vi "PrepareRollToPassRollerGoToTactic.vi"(7 "first call":bool, 8 "error in (no error)":errorcluster, 9 "Robot":refnum<class "Robot.lvclass">, 10 "Game in":refnum<class "Game.lvclass">, 11 "PrepareRollToPassRollerGoToTactic in":refnum<class "PrepareRollToPassRollerGoToTactic.lvclass">) -> (0 "error out":errorcluster, 2 "Robot out":refnum<class "Robot.lvclass">, 3 "PrepareRollToPassRollerGoToTactic out":refnum<class "PrepareRollToPassRollerGoToTactic.lvclass">)   [LabVIEW 2023, in "PrepareRollToPassRollerGoToTactic.lvclass"]
uses:
  PrepareRollToPassRollerGoToTactic.lvclass
  Robot_class/Robot.lvclass
  Game_class/Game.lvclass
  Robot_class/tactics.ctl
  Tactic_class/Tactic.lvclass/Tactic.ctl
  Skillbook_class/Skillbook.lvclass/Skillbook.ctl
  Robot_class/Robot.lvclass/Robot.ctl
  Object_class/Object.lvclass/Object.ctl
  Game_class/Game.lvclass/Game.ctl
  Parameters_class/Parameters.lvclass/Parameters.ctl
  Team_class/Team.lvclass/Team.ctl
  PrepareRollToPassRollerGoToTactic.lvclass/PrepareRollToPassRollerGoToTactic.ctl
  <vilib>/Analysis/_algsub.llb/Real Vector Norm.vi
  Game_class/Read Parameters.lvclass.vi
  Game_class/Read Utilities.lvclass.vi
  Game_class/Read OffensiveTeam.vi
  Team_class/Read RobotRef.vi
  Parameters_class/Read AttakingOurselves.vi
  Game_class/Read BallRef.vi
  Object_class/Read x.vi
  Object_class/Read y.vi
  Robot_class/Read id.vi
  Skillbook_class/Read GoToSkill.vi
  Tactic_class/Read Skillbook.vi
  Robot_class/Write tactic.vi
  Write States.vi
  Ball_class/Ball.lvclass
  Ally_class/Ally.lvclass
  Skillbook_class/Skillbook.lvclass
  Parameters_class/Parameters.lvclass
  Utilities_class/Utilities.lvclass
  GoToSkill_class/GoToSkill.lvclass
  <vilib>/Analysis/NI_AALPro.lvlib
panel:
  out "x .or. y?":bool
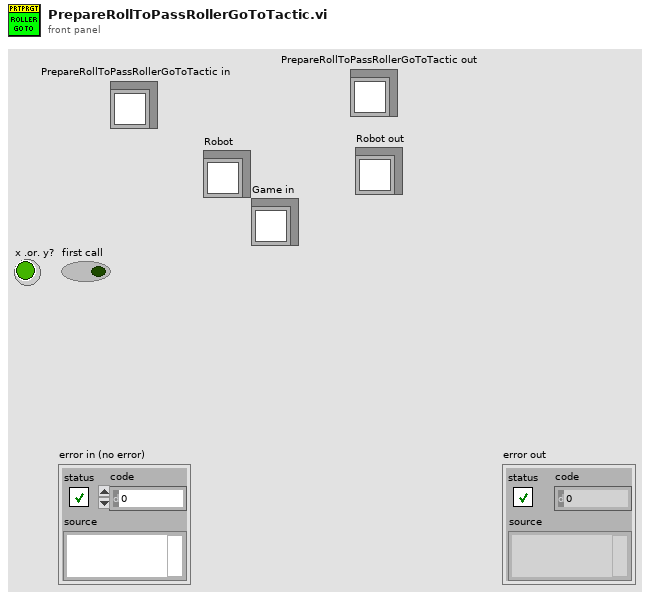
[diagram p1: front panel]
types:
  T1 = typedef "tactics.ctl" = enum16{"ReceivePassInFuturePoint", "Roller", "PrepareRollToPassRollerGoTo", "PrepareRollToPassReceiverGoTo", "WaitRoll", "PositionToRoll", "PenaltyAttacker", "PassObserver", "PenaltyDefense", "TableReceiverTactic", "Test", "DefendGoal", "Marker", "FollowAttacker", "DefendArea", "Shoot", "AttackerAimGoal", "AttackerBallOutOfField", "AttackerBlock", "AttackerStop", "Duelist", "Halt", "ZigZag", "GoTo", "Timeout", "KickToPassReceiver", "PositionToReceivePass", "DefendAreaVSS", "DefendGoalVSS", "KickVSS", "AttackVSS", "DispBallVSS", "PenaltyAttackVSS", "WaitPass"}
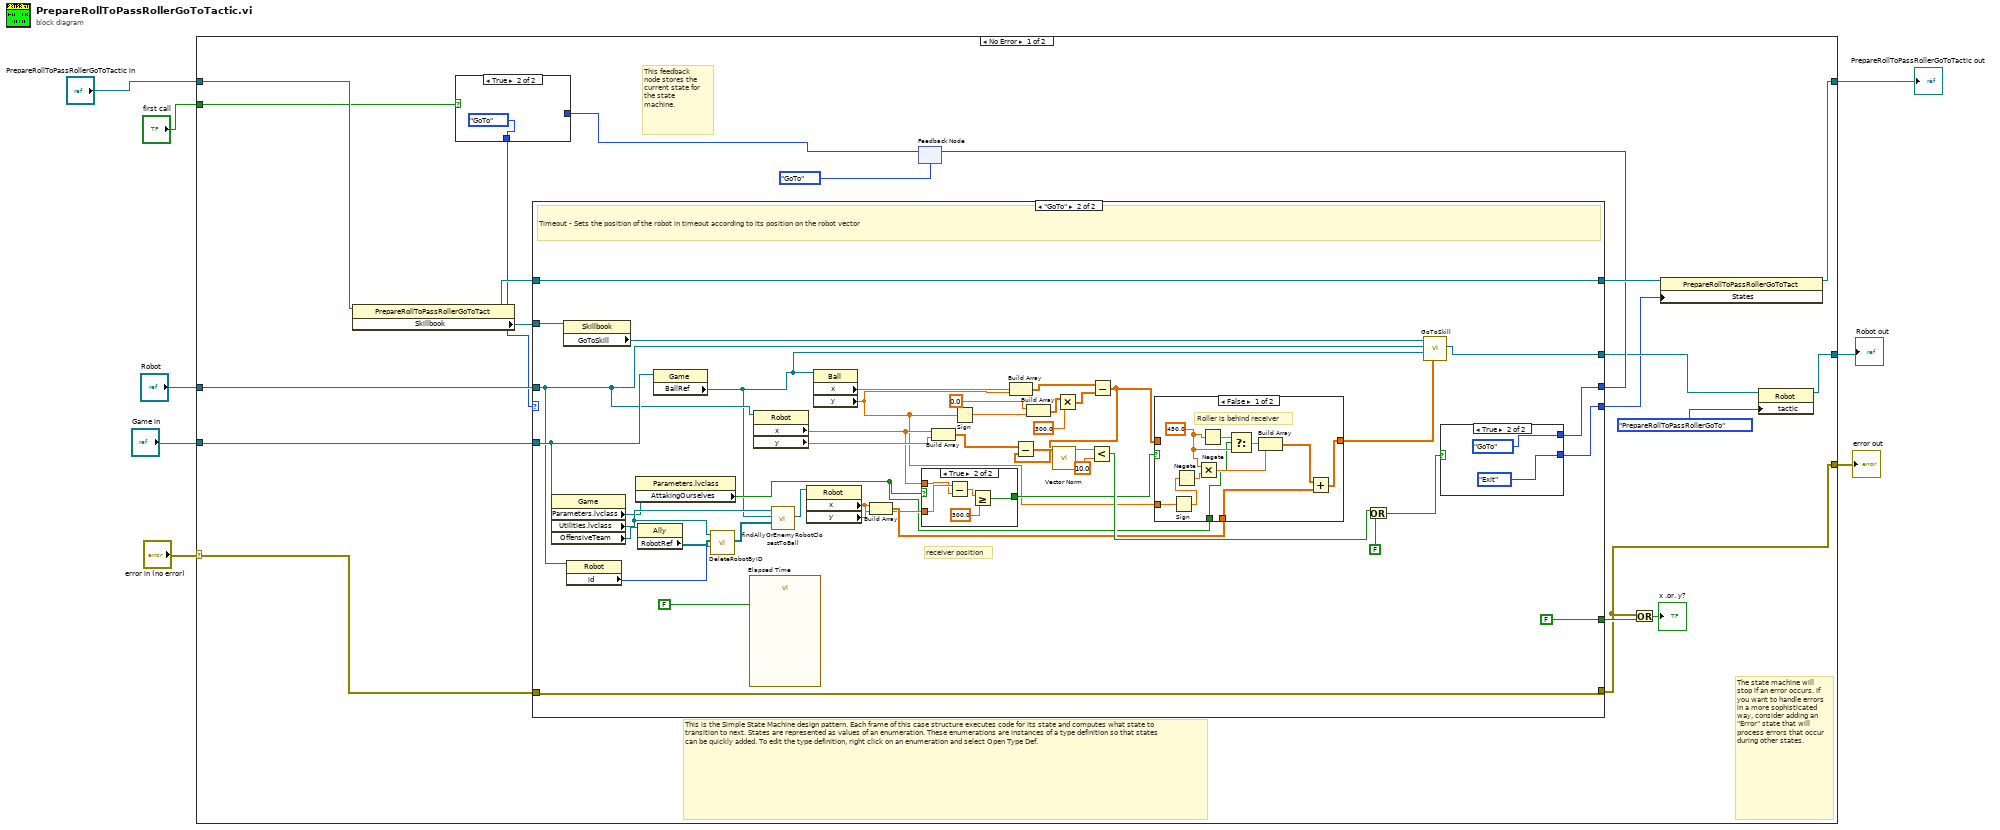
[diagram p0: block diagram]
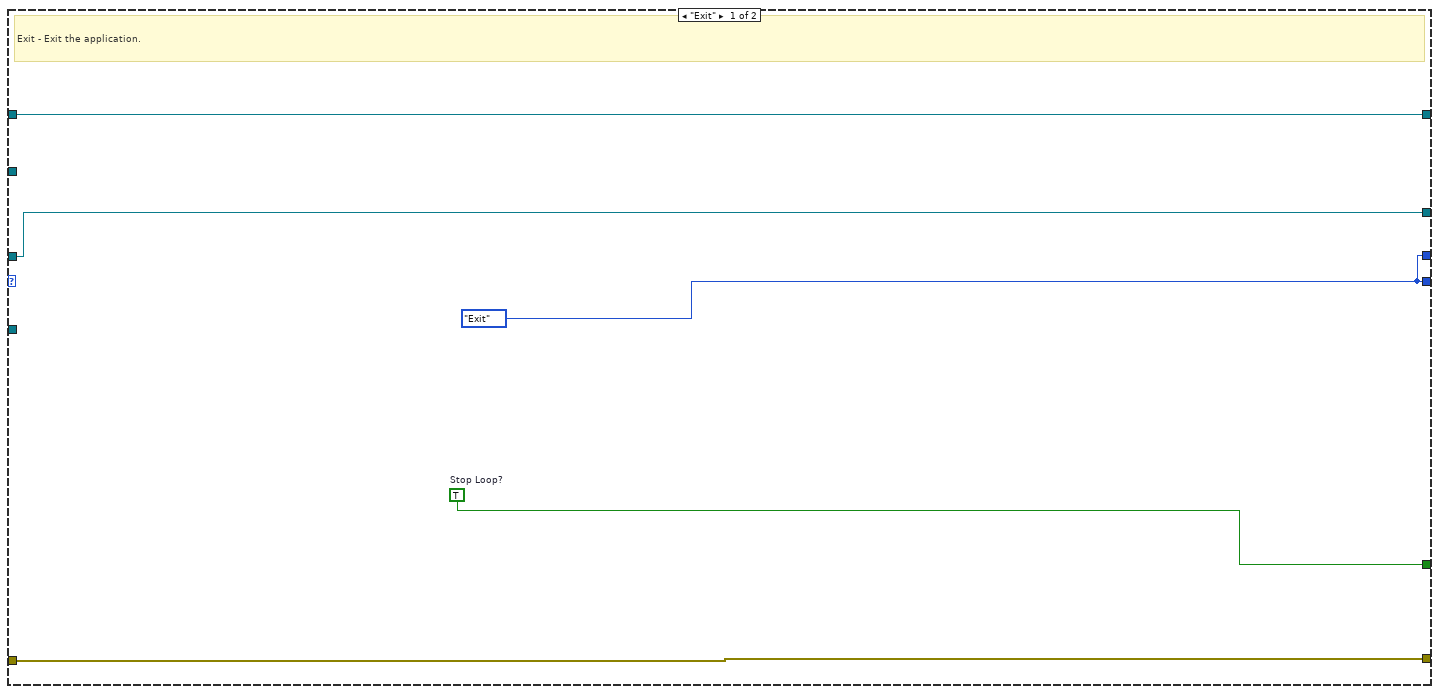
[diagram p3: hidden frame]
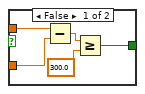
[diagram p4: hidden frame]
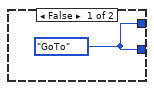
[diagram p6: hidden frame]
diagram:
  n1 = case shown="No Error" "error in (no error)" {
    selector: "error in (no error)" -> [w23 w106]
    tunnel: [w24 w106] -> w7
    tunnel: [w21 w105] -> w1
    tunnel: "PrepareRollToPassRollerGoToTactic in" -> [w22 w105]
    tunnel: "Game in" -> [w19 _]
    tunnel: "Robot" -> [w18 w104]
    tunnel: [w11 w104] -> w5
    tunnel: "first call" -> [w16 _]
    frame No Error {
      # "The state machine will stop if an error occurs. If you want to handle errors in a more sophisticated way, consider adding an \"Error\" state that will process errors that occur during other states."
      # "This feedback node stores the current state for the state machine."
      # "This is the Simple State Machine design pattern. Each frame of this case structure executes code for its state and computes what state to transition to next. States are represented as values of an enumeration. These enumerations are instances of a type definition so that states can be quickly added. To edit the type definition, right click on an enumeration and select Open Type Def."
      n2 = property class="PrepareRollToPassRollerGoToTact"(reference=w22) -> (reference out=w20:refnum<class "PrepareRollToPassRollerGoToTactic.lvclass">, "Skillbook"=w26:refnum<class "Skillbook.lvclass">)  [unwired: 1 in, 1 out]
      n3 = feedback #1(enum16{"GoTo", "Exit"}."GoTo" ("States")) -> (w14:enum16{"GoTo", "Exit"})
      n4 = case shown="True" w16 {
        tunnel: [w29 enum16{"GoTo", "Exit"}."GoTo" ("States")] -> w15
        tunnel: w14 -> [w29 _]
        frame False {
        }
        frame True {
        }
      }
      n5 = case shown="\"GoTo\"" w15 {
        tunnel: [w31 w74] -> w10
        tunnel: [w35 FALSE ("Stop Loop?")] -> w28
        tunnel: w23 -> [w34 w77]
        tunnel: [w34 w77] -> w24
        tunnel: w26 -> [_ w76]
        tunnel: w18 -> [w33 w45]
        tunnel: [w33 w57] -> w12
        tunnel: [w32 w75] -> w25
        tunnel: w20 -> [w32 w75]
        tunnel: w19 -> [_ w55]
        tunnel: [w31 w73] -> w17
        frame "Exit" {
          w31 = enum16{"GoTo", "Exit"}."Exit" ("States")
          w35 = TRUE  # Stop Loop?
          # "Exit - Exit the application."
        }
        frame "GoTo" {
          # "receiver position"
          # "Timeout - Sets the position of the robot in timeout according to its position on the robot vector"
          n6 = property class="Game"(reference=w55) -> ("Parameters.lvclass"=w38:refnum<class "Parameters.lvclass">, "Utilities.lvclass"=w39:refnum<class "Utilities.lvclass">, "OffensiveTeam"=w54:refnum<class "Ally.lvclass">)  [unwired: 1 in, 2 out]
          n7 = property class="Skillbook"(reference=w76) -> ("GoToSkill"=w72:refnum<class "GoToSkill.lvclass">)  [unwired: 1 in, 2 out]
          n8 = property class="Robot"(reference=w45) -> ("id"=w52:i32)  [unwired: 1 in, 2 out]
          n9 = property class="Parameters.lvclass"(reference=w38) -> ("AttakingOurselves"=w37:bool)  [unwired: 1 in, 2 out]
          n10 = property class="Ally"(reference=w54) -> ("RobotRef"=w53:refnum<class "Robot.lvclass">[])  [unwired: 1 in, 2 out]
          n11 = property class="Game"(reference=w55) -> ("BallRef"=w36:refnum<class "Ball.lvclass">)  [unwired: 1 in, 2 out]
          n12 = call-dynamic "DeleteRobotByID.vi"("id"=w52, "RobotRef"=w53, "Utilities in"=w39) -> ("RobotRef out"=w51:refnum<class "Robot.lvclass">[])  [unwired: 6 in, 2 out]
          n13 = call "Elapsed Time"("Auto Reset"=FALSE) -> ()  [unwired: 11 in, 8 out]
          n14 = property class="Robot"(reference=w45) -> ("x"=w43:dbl, "y"=w71:dbl)  [unwired: 1 in, 2 out]
          n15 = call "findAllyOrEnemyRobotClosestToBall.vi"("Ally/Enemy Robots"=w51, "Ball"=w36, "Utilities in"=w39) -> ("Robot"=w49:refnum<class "Robot.lvclass">)  [unwired: 5 in, 3 out]
          n16 = property class="Robot"(reference=w49) -> ("x"=w42:dbl, "y"=w48:dbl)  [unwired: 1 in, 2 out]
          n17 = property class="Ball"(reference=w36) -> ("x"=w65:dbl, "y"=w40:dbl)  [unwired: 1 in, 2 out]
          n18 = Build Array(w42, w48) -> (w46:dbl[])
          n19 = case shown="True" w37 {
            tunnel: w43 -> [w83 w84]
            tunnel: w42 -> [w82 w85]
            tunnel: [w79 w87] -> w41
            frame False {
              n20 = Subtract(x=w83, y=w82) -> (x-y=w81:dbl)
              n21 = Greater Or Equal?(x=w81, y=300.0) -> (x >= y?=w79:bool)
            }
            frame True {
              n22 = Subtract(x=w85, y=w84) -> (x-y=w88:dbl)
              n23 = Greater Or Equal?(x=w88, y=300.0) -> (x >= y?=w87:bool)
            }
          }
          n24 = Build Array(w43, w71) -> (w50:dbl[])
          n25 = Sign(1:w40) -> (0:w63:dbl)
          n26 = Build Array(w65, w40) -> (w64:dbl[])
          n27 = Build Array(0.0 ("element"), w63) -> (w60:dbl[])
          n28 = Multiply(x=w60, y=300.0 ("element")) -> (x*y=w61:dbl[])
          n29 = Subtract(x=w64, y=w61) -> (x-y=w47:dbl[])
          n30 = Subtract(x=w50, y=w47) -> (x-y=w70:dbl[])
          n31 = call-poly <vilib>:"Vector Norm.vi"("Input Vector"=w70) -> ("norm"=w69:dbl)  [unwired: 9 in, 1 out]
          n32 = Less?(x=w69, y=10.0) -> (x < y?=w56:bool)
          n33 = case shown="False" w41 {
            tunnel: [w98 w100] -> w44
            tunnel: w47 -> [_ w100]
            tunnel: w46 -> [w99 _]
            tunnel: w40 -> [w97 _]
            tunnel: w37 -> [w89 _]
            frame False {
              w90 = 450.0
              # "Roller is behind receiver"
              n34 = Sign(1:w97) -> (0:w96:dbl)
              n35 = Negate(x=w96) -> (-x=w95:dbl)
              n36 = Multiply(x=w90, y=w95) -> (x*y=w94:dbl)
              n37 = Negate(x=w90) -> (-x=w92:dbl)
              n38 = Select(t=w92, s=w89, f=w90) -> (s? t:f=w91:dbl)
              n39 = Build Array(w91, w94) -> (w93:dbl[])
              n40 = Add(x=w93, y=w99) -> (x+y=w98:dbl[])
            }
            frame True {
              # "Roller is already ahead receiver"
            }
          }
          n41 = Or(x=w56, y=FALSE) -> (x .or. y?=w66:bool)
          n42 = call "GoToSkill.vi"("Position"=w44, "BallRef"=w36, "Robot in"=w45, "GoToSkill in"=w72) -> ("Robot out"=w57:refnum<class "Robot.lvclass">)  [unwired: 5 in, 2 out]
          n43 = case shown="True" w66 {
            tunnel: [w101 enum16{"GoTo", "Exit"}."Exit" ("States")] -> w74
            tunnel: [w101 enum16{"GoTo", "Exit"}."GoTo" ("States")] -> w73
            frame False {
              w101 = enum16{"GoTo", "Exit"}."GoTo" ("States")
            }
            frame True {
            }
          }
        }
      }
      n44 = feedback-in #1(w17) -> ()
      n45 = Or(x=w24, y=w28) -> (x .or. y?=→"x .or. y?":bool)
      n46 = property class="PrepareRollToPassRollerGoToTact"(reference=w25, "States"=w10) -> (reference out=w21:refnum<class "PrepareRollToPassRollerGoToTactic.lvclass">)  [unwired: 1 in, 1 out]
      n47 = property class="Robot"(reference=w12, "tactic"=tactics."PrepareRollToPassRollerGoTo") -> (reference out=w11:refnum<class "Robot.lvclass">)  [unwired: 1 in, 1 out]
    }
    frame Error {
    }
  }
  "error out" <- w7
  "Robot out" <- w5
  "PrepareRollToPassRollerGoToTactic out" <- w1
